vi "CAPTH-Find Threshold.vi"(0 "tone":dbl[](array[numeric]), 1 "Channels":cluster{"Output":u16, "Input":u16}, 2 "IPC":T2, 5 "runtime":T3, 7 "dB refs":refnum<vi>[](array[refnum]), 9 "Response":T4={"Averages (3dB steps)"=12, "Time Window (ms)"=8.5, "dt (us)"=10.0, "Grass gain"=1000.0, "CRITERION (mV)"=5.0, "CEILING (dB atten)"=60.0, "Use previous"=FALSE, "Save avgs"=FALSE, "Save raw"=FALSE, "Save history"=FALSE, "CEILING (dB SPL)"=6.0} {"CRITERION (mV)" format="%.2f"; "Time Window (ms)" format="%.2f"}, 11 "error in (no error)":errorcluster, 12 "Start atten":dbl, 13 "stimcon":T1) -> (3 "Abort":bool, 4 "runtime out":T3, 6 "Threshold":dbl, 15 "error out":errorcluster)   [LabVIEW 2020]
uses:
  Typedefs/CAPTH-Response.ctl
  Typedefs/CAPTH-Runtime.ctl
  Typedefs/CAPTH-IPC.ctl
  Typedefs/CAPTH-Start Data.ctl
  Typedefs/CAPTH-Parameters.ctl
  Typedefs/CAPTH-Stimulus.ctl
  Typedefs/CAPTH-Analysis Message.ctl
  Typedefs/CAPTH-Analysis Action.ctl
  Typedefs/CAPTH-StimCon.ctl
  Typedefs/CAPTH-Analysis Data Properties.ctl
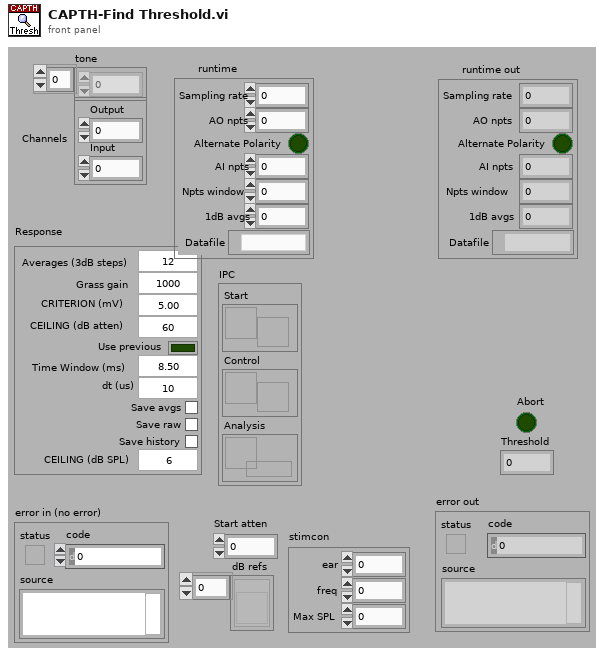
[diagram p1: front panel]
types:
  T1 = typedef "CAPTH-StimCon.ctl" = cluster{"ear":i32, "freq":i32, "Max SPL":dbl}
  T2 = typedef "CAPTH-IPC.ctl" = cluster{"Start":refnum<notifier>, "Control":refnum<notifier>, "Analysis":refnum<queue>}
  T3 = typedef "CAPTH-Runtime.ctl" = cluster{"Sampling rate":dbl, "AO npts":i32, "Alternate Polarity":bool, "AI npts":i32, "Npts window":i32, "1dB avgs":i32, "Datafile":path}
  T4 = typedef "CAPTH-Response.ctl" = cluster{"Averages (3dB steps)":i32, "Time Window (ms)":dbl, "dt (us)":dbl, "Grass gain":dbl, "CRITERION (mV)":dbl, "CEILING (dB atten)":dbl, "Use previous":bool, "Save avgs":bool, "Save raw":bool, "Save history":bool, "CEILING (dB SPL)":dbl}
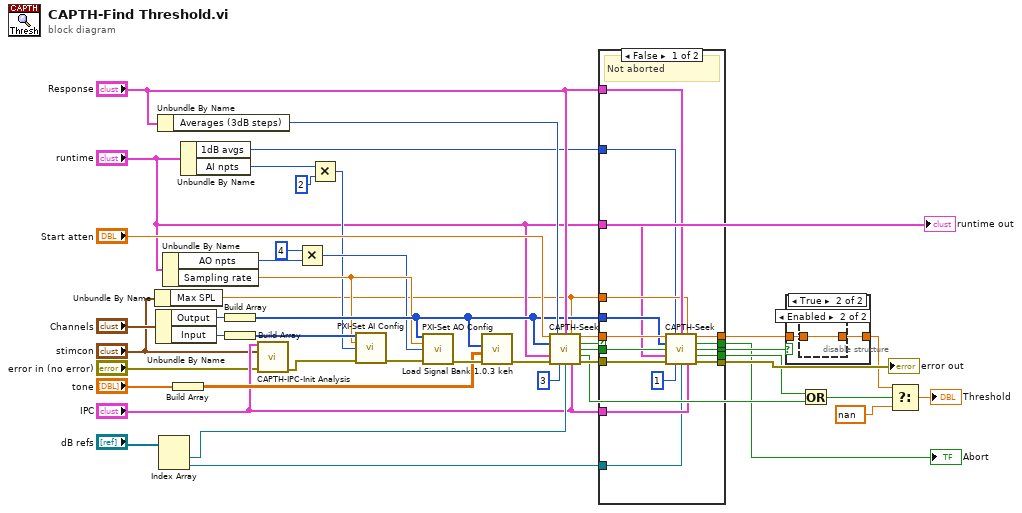
[diagram p0: block diagram]
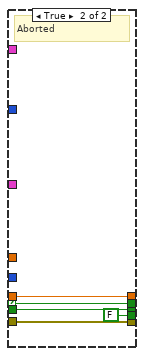
[diagram p2: hidden frame]
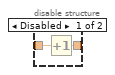
[diagram p4: hidden frame]
diagram:
  n1 = Unbundle By Name("stimcon") -> ("Max SPL"=w1:dbl)
  n2 = Unbundle By Name("Channels") -> ("Output"=w32:u16, "Input"=w43:u16)
  n3 = Unbundle By Name("Response") -> ("Averages (3dB steps)"=w33:i32)
  n4 = Index Array(array="dB refs") -> (element #1=w8:refnum<vi>, element #2=w7:refnum<vi>)  [unwired: 2 in]
  n5 = Unbundle By Name("runtime") -> ("AO npts"=w25:i32, "Sampling rate"=w26:dbl)
  n6 = Build Array("tone") -> (w20:dbl[][])
  n7 = Unbundle By Name("runtime") -> ("1dB avgs"=w12:i32, "AI npts"=w13:i32)
  n8 = Build Array(w32) -> (w27:u16[])
  n9 = Build Array(w43) -> (w28:u16[])
  n10 = call "CAPTH-IPC-Init Analysis.vi"("IPC"="IPC", "stimcon"="stimcon", "error in (no error)"="error in (no error)") -> ("error out"=w3:errorcluster)  [unwired: 12 in]
  n11 = Multiply(x=4, y=w25) -> (x*y=w23:i32)
  n12 = Multiply(x=w13, y=2) -> (x*y=w21:i32)
  n13 = call "PXI-Set AI Config.vi"("AI Channels"=w28, "Sampling Rate (Hz)"=w26, "Buffer Size"=w21, "error in (no error)"=w3) -> ("error out"=w44:errorcluster)  [unwired: 11 in]
  n14 = call "PXI-Set AO Config.vi"("AO Channels"=w27, "Sampling Rate (Hz)"=w26, "Buffer Size"=w23, "error in (no error)"=w44) -> ("error out"=w42:errorcluster)  [unwired: 11 in]
  n15 = call "Load Signal Bank 1.0.3 keh.vi"("error in (no error)"=w42, "Input array"=w20, "Active AO Array"=w27) -> ("error out"=w39:errorcluster)  [unwired: 6 in, 2 out]
  n16 = call "CAPTH-Seek.vi"("Start atten"="Start atten", "Navg"=w33, "Response"="Response", "Max SPL"=w1, "AO channels"=w27, "Runtime"="runtime", "error in (no error)"=w39, "step size"=3, "dB ref"=w8, "IPC"="IPC") -> ("End atten"=w36:dbl, "abort"=w6:bool, "suprathreshold out"=w31:bool, "any supra"=w18:bool, "error out"=w40:errorcluster)  [unwired: 1 in]
  n17 = case shown="False" w6 {
    selector: w6 -> [_ w65]
    tunnel: w40 -> [w61 w63]
    tunnel: [w60 w63] -> w38
    tunnel: w36 -> [w59 w66]
    tunnel: "Response" -> [w58 _]
    tunnel: w31 -> [w57 w64]
    tunnel: [w55 w64] -> w30
    tunnel: [w54 w66] -> w29
    tunnel: w27 -> [w53 _]
    tunnel: w1 -> [w52 _]
    tunnel: [w51 FALSE ("any supra")] -> w19
    tunnel: w12 -> [w50 _]
    tunnel: "runtime" -> [w49 _]
    tunnel: [w48 w65] -> w10
    tunnel: "IPC" -> [w47 _]
    tunnel: w7 -> [w46 _]
    frame False {
      # "Not aborted"
      n18 = call "CAPTH-Seek.vi"("Start atten"=w59, "Navg"=w50, "Response"=w58, "Max SPL"=w52, "AO channels"=w53, "suprathreshold?"=w57, "Runtime"=w49, "error in (no error)"=w61, "step size"=1, "dB ref"=w46, "IPC"=w47) -> ("End atten"=w54:dbl, "abort"=w48:bool, "suprathreshold out"=w55:bool, "any supra"=w51:bool, "error out"=w60:errorcluster)
    }
    frame True {
      # "Aborted"
    }
  }
  "error out" <- w38
  "Abort" <- w10
  n19 = case shown="True" w30 {
    tunnel: w29 -> [w67 w69]
    tunnel: [w67 w68] -> w15
    frame False {
    }
    frame True {
      n20 = disable-structure shown="Enabled" {
        disable-tunnel: w69 -> [w71 w72]
        disable-tunnel: [w70 w72] -> w68
        frame Disabled {
          n21 = Increment(x=w71) -> (x+1=w70:dbl)
        }
        frame Enabled {
        }
      }
    }
  }
  n22 = Or(x=w19, y=w18) -> (x .or. y?=w17:bool)
  n23 = Select(t=w15, s=w17, f=nan) -> (s? t:f=→"Threshold":dbl)
  "runtime out" <- "runtime"
